vi "Default TextManager Object.vi"(11 "CfgManager.Text in":refnum<class "ConfigManager.Text.lvclass">) -> (3 "CfgManager.Text out":refnum<class "ConfigManager.Text.lvclass">)   [LabVIEW 2013, in "CfgManager.Text.lvlib" / "ConfigManager.Text.lvclass"]
uses:
  ConfigManager.Text.lvclass
  FileHeader/FileHeader.lvclass
  FileSignature/FileSignature.lvclass
  <vilib>/LabVIEW Open Source Project/Unicity/Delimiter/Delimiter.lvclass
  <vilib>/LabVIEW Open Source Project/Unicity/Delimiter/Delimiters List.ctl
  Manager/ConfigManager.lvclass
  <vilib>/LabVIEW Open Source Project/Serializer/Serializer.PlainText/Serializer.PlainText.lvclass
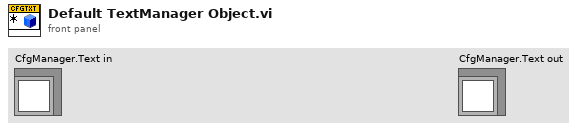
[diagram p1: front panel]
types:
  T1 = typedef "Delimiter.lvclass/Delimiters List.ctl" = enum16{"Default", "dot (.)", "colon (:)", "double-colon (::)", "semi-colon (;)", "underscore (_)", "double underscore (__)", "dash (-)", "double dash (--)", "backslash (\\)", "vertical bar (|)", "forward slash (/)", "chevron (>)", "double-chevron (>>)", "arrow (->)", "comma (,)", "arobas (@)", "ampersand (&)", "other"}
  T2 = typedef "CfgManager.Text.lvlib/ConfigManager.Text.lvclass/Configuration -- Cluster.ctl" = cluster{"FileHeader":refnum<class "FileHeader.lvclass">, "FileSignature":refnum<class "FileSignature.lvclass">, "Section Delimiter":refnum<class "Delimiter.lvclass">, "Key-Value Separator":refnum<class "Delimiter.lvclass">}
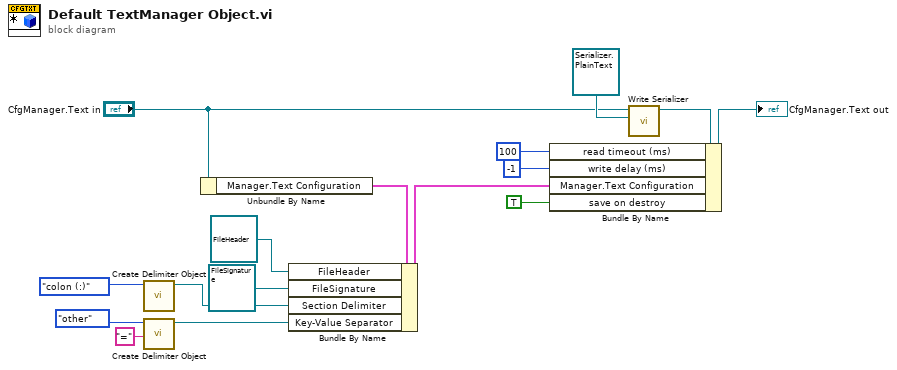
[diagram p0: block diagram]
diagram:
  n1 = call <vilib>:"Create Delimiter Object.vi"("Delimiter"=Delimiters_List."colon (:)") -> ("Delimiter"=w5:refnum<class "Delimiter.lvclass">)  [unwired: 10 in]
  n2 = call <vilib>:"Create Delimiter Object.vi"("Other"="=", "Delimiter"=Delimiters_List."other") -> ("Delimiter"=w4:refnum<class "Delimiter.lvclass">)  [unwired: 9 in]
  n3 = Unbundle By Name("CfgManager.Text in") -> ("Manager.Text Configuration"=w9:T2)
  n4 = Bundle By Name(cluster=w9, "FileHeader"=refnum<class "FileHeader.lvclass"> refnum, "FileSignature"=refnum<class "FileSignature.lvclass"> refnum, "Section Delimiter"=w5, "Key-Value Separator"=w4) -> (w13:T2)
  n5 = call "Write Serializer.vi"("Serializer"=refnum<class "Serializer.PlainText.lvclass"> refnum, "ConfigManager in"="CfgManager.Text in") -> ("ConfigManager out"=w10:refnum<class "ConfigManager.Text.lvclass">)  [unwired: 9 in]
  n6 = Bundle By Name(cluster=w10, "read timeout (ms)"=100, "write delay (ms)"=-1, "Manager.Text Configuration"=w13, "save on destroy"=TRUE) -> (→"CfgManager.Text out":refnum<class "ConfigManager.Text.lvclass">)
